vi "Close Session.vi"(6 "version (no change)":T1, 8 "error in (no error)":errorcluster, 10 "write file if changed (T)":bool=TRUE, 11 "configuration session":refnum<class "Configuration Session.lvclass">) -> (0 "error out":errorcluster, 3 "file path":path)   [LabVIEW 2017, in "DSF Core.lvlib" / "Configuration Session.lvclass"]
doc: "Writes data to the platform-independent configuration file identified by <B>dsf refnum</B> and then closes the reference to that file."
uses:
  Configuration Session.lvclass
  Typedefs/DSF Version Info.ctl
  Configuration Session.lvclass/Configuration Session.ctl
  DSF Core.lvlib
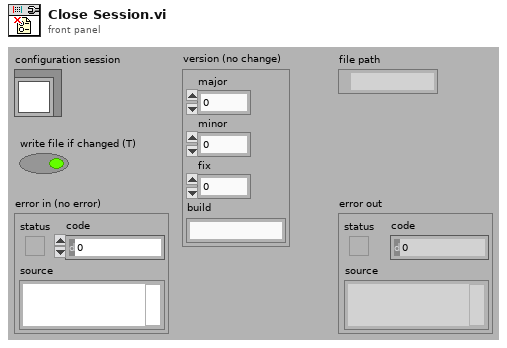
[diagram p1: front panel]
types:
  T1 = typedef "DSF Core.lvlib/DSF Version Info.ctl" = cluster{"major":u32, "minor":u32, "fix":u32, "build":string}
  T2 = cluster{"major":bool, "minor":bool, "fix":bool, "build":bool}
  T3 = typedef "DSF Core.lvlib/Configuration Session.lvclass/DSF Config Data Ref.ctl" = refnum<data-value>
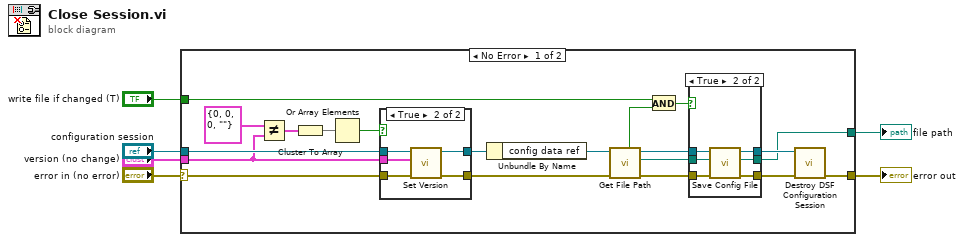
[diagram p0: block diagram]
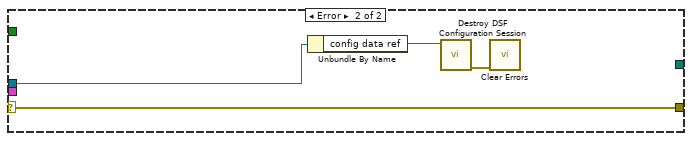
[diagram p4: hidden frame]
diagram:
  n1 = case shown="No Error" "error in (no error)" {
    selector: "error in (no error)" -> [w14 w46]
    tunnel: "configuration session" -> [w15 w44]
    tunnel: "write file if changed (T)" -> [w26 _]
    tunnel: [w25 w46] -> w4
    tunnel: [w16 _] -> w3
    tunnel: "version (no change)" -> [w8 _]
    frame No Error {
      n2 = Not Equal?(x=T1 {"major"=0, "minor"=0, "fix"=0, "build"=""}, y=w8) -> (x != y?=w11:T2)
      n3 = Cluster To Array(cluster=w11) -> (array=w9:bool[])
      n4 = Or Array Elements(Boolean array=w9) -> (logical OR=w7:bool)
      n5 = case shown="True" w7 {
        tunnel: w15 -> [w28 w33]
        tunnel: w14 -> [w27 w32]
        tunnel: [w28 w31] -> w13
        tunnel: [w27 w30] -> w12
        tunnel: w8 -> [_ w29]
        frame False {
        }
        frame True {
          n6 = call "Set Version.vi"("error in (no error)"=w32, "version"=w29, "configuration session in"=w33) -> ("error out"=w30:errorcluster, "configuration session out"=w31:refnum<class "Configuration Session.lvclass">)  [unwired: 7 in]
        }
      }
      n7 = Unbundle By Name(w13) -> ("config data ref"=w17:T3)
      n8 = call "Get File Path.vi"("error in (no error)"=w12, "DSF Configuration Reference in"=w17) -> ("error out"=w19:errorcluster, "file path"=w18:path, "DSF Configuration Reference out"=w23:T3, "need update"=w20:bool)  [unwired: 1 in, 5 out]
      n9 = And(x=w26, y=w20) -> (x .and. y?=w24:bool)
      n10 = case shown="True" w24 {
        tunnel: w19 -> [w36 w42]
        tunnel: w23 -> [w35 w37]
        tunnel: [w36 w41] -> w21
        tunnel: [w35 w40] -> w22
        tunnel: w18 -> [w34 w39]
        tunnel: [w34 w38] -> w16
        frame False {
        }
        frame True {
          n11 = call "Save Config File.vi"("error in (no error)"=w42, "file path"=w39, "DSF Configuration Reference in"=w37) -> ("error out"=w41:errorcluster, "file path out"=w38:path, "DSF Configuration Reference out"=w40:T3)  [unwired: 6 out]
        }
      }
      n12 = call "Destroy DSF Configuration Session.vi"("error in (no error)"=w21, "config data ref"=w22) -> ("error out"=w25:errorcluster)  [unwired: 9 in]
    }
    frame Error {
      n13 = Unbundle By Name(w44) -> ("config data ref"=w43:T3)
      n14 = call "Destroy DSF Configuration Session.vi"("config data ref"=w43) -> ("error out"=w45:errorcluster)  [unwired: 10 in]
      n15 = call <vilib>:"Clear Errors.vi"("error in (no error)"=w45) -> ()  [unwired: 5 in, 2 out]
    }
  }
  "error out" <- w4
  "file path" <- w3
